vi "ma_sml_RRC Power Spectrum for each Channel.vi"(8 "beta":dbl, 9 "n":i32, 10 "T":dbl, 11 "df":dbl) -> (3 "RRC power spectrum":dbl[](array[numeric]))   [LabVIEW 2020, in "NI_MAPro.lvlib"]
uses:
  NI_MAPro.lvlib
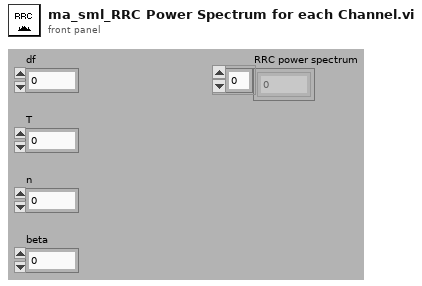
[diagram p1: front panel]
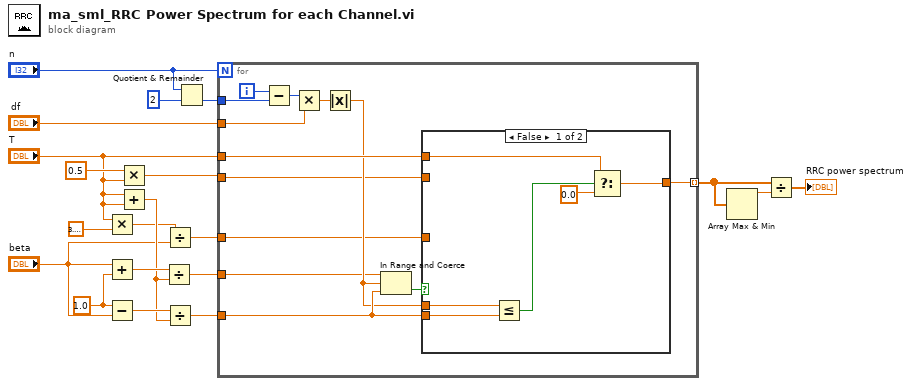
[diagram p0: block diagram]
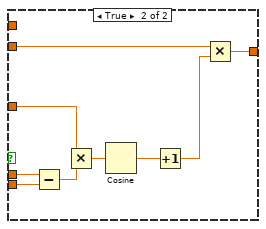
[diagram p2: hidden frame]
diagram:
  w11 = 1.0 ("x")
  n1 = Multiply(x="T", y=3.141592653589793) -> (x*y=w1:dbl)
  n2 = Add(x="beta", y=w11) -> (x+y=w15:dbl)
  n3 = Subtract(x=w11, y="beta") -> (x-y=w16:dbl)
  n4 = Multiply(x=0.5, y="T") -> (x*y=w6:dbl)
  n5 = Add(x="T", y="T") -> (x+y=w12:dbl)
  n6 = Divide(x=w15, y=w12) -> (x/y=w14:dbl)
  n7 = Divide(x=w1, y="beta") -> (x/y=w7:dbl)
  n8 = Divide(x=w16, y=w12) -> (x/y=w13:dbl)
  n9 = Quotient & Remainder(x="n", y=2) -> (floor(x/y)=w4:i32)  [unwired: 1 out]
  n10 = for {
    N: "n" -> [_]
    tunnel: "T" -> [w33]
    tunnel: [w32] -> w19 mode=indexing
    tunnel: "df" -> [w31]
    tunnel: w14 -> [w23]
    tunnel: w13 -> [w29]
    tunnel: w7 -> [w25]
    tunnel: w6 -> [w24]
    tunnel: w4 -> [w21]
    i -> [w22]
    n11 = Subtract(x=w22, y=w21) -> (x-y=w28:i32)
    n12 = Multiply(x=w28, y=w31) -> (x*y=w27:dbl)
    n13 = Absolute Value(x=w27) -> (abs(x)=w26:dbl)
    n14 = In Range and Coerce(upper limit=w23, x=w26, lower limit=w29) -> (In Range?=w30:bool)  [unwired: 1 out]
    n15 = case shown="False" w30 {
      tunnel: w26 -> [w36 w48]
      tunnel: w33 -> [w38 _]
      tunnel: w29 -> [w34 w47]
      tunnel: [w37 w44] -> w32
      tunnel: w25 -> [_ w42]
      tunnel: w24 -> [_ w43]
      frame False {
        n16 = Less Or Equal?(x=w36, y=w34) -> (x <= y?=w35:bool)
        n17 = Select(t=w38, s=w35, f=0.0) -> (s? t:f=w37:dbl)
      }
      frame True {
        n18 = Subtract(x=w48, y=w47) -> (x-y=w41:dbl)
        n19 = Multiply(x=w42, y=w41) -> (x*y=w46:dbl)
        n20 = Cosine(x=w46) -> (cos(x)=w45:dbl)
        n21 = Increment(x=w45) -> (x+1=w40:dbl)
        n22 = Multiply(x=w43, y=w40) -> (x*y=w44:dbl)
      }
    }
  }
  n23 = Array Max & Min(array=w19) -> (max value=w20:dbl)  [unwired: 3 out]
  n24 = Divide(x=w19, y=w20) -> (x/y=→"RRC power spectrum":dbl[])
